vi "writeToXML.vi"(8 "error in (no error)":errorcluster, 10 "ClassLabel":string, 11 "TCSActiveOpticsCommand in":refnum<class "TCSActiveOpticsCommand.lvclass">) -> (0 "error out":errorcluster, 2 "XML out":string, 3 "TCSActiveOpticsCommand out":refnum<class "TCSActiveOpticsCommand.lvclass">)   [LabVIEW 2014, in "TCSDataDefinitions.lvlib" / "TCSActiveOpticsCommand.lvlib" / "TCSActiveOpticsCommand.lvclass"]
uses:
  TCSActiveOpticsCommand.lvclass
  TCSCommand/TCSCommand/TCSCommand.lvclass
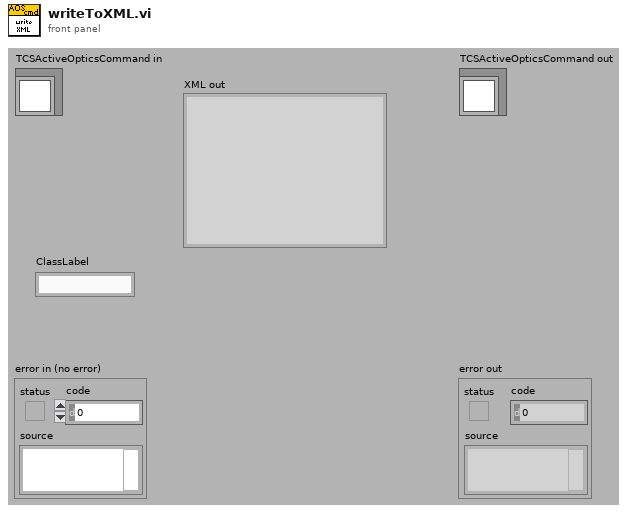
[diagram p1: front panel]
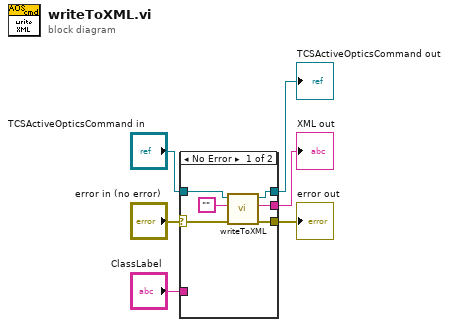
[diagram p0: block diagram]
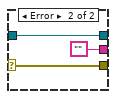
[diagram p2: hidden frame]
diagram:
  n1 = case shown="No Error" "error in (no error)" {
    selector: "error in (no error)" -> [w8 w15]
    tunnel: [w7 w15] -> w5
    tunnel: [w11 w14] -> w3
    tunnel: "TCSActiveOpticsCommand in" -> [w12 w14]
    tunnel: [w9 ""] -> w2
    tunnel: "ClassLabel" -> [_ _]
    frame No Error {
      n2 = call-parent "writeToXML.vi"("error in (no error)"=w8, "Class Label"="", "TCSCommand in"=w12) -> ("error out"=w7:errorcluster, "XML out"=w9:string, "TCSCommand out"=w11:refnum<class "TCSActiveOpticsCommand.lvclass">)  [unwired: 6 in]
    }
    frame Error {
    }
  }
  "error out" <- w5
  "TCSActiveOpticsCommand out" <- w3
  "XML out" <- w2
